vi "Add Acyclic Frame Triggers in Section.vi"(8 "error in":errorcluster, 10 "acyclic frames":T1[](array[typedef]), 11 "acyclic frames section":T2=18446744073709551615 format="%.0x") -> (0 "error out":errorcluster, 3 "acyclic frames section out":T2=18446744073709551615 format="%.0x")   [LabVIEW 2020, in "AIM MIL-STD-1553 Scripting.lvlib"]
doc: "Adds an Acyclic Frame Trigger for each element in <b>acyclic frames</b> to the <b>acyclic frames section</b>."
uses:
  AIM MIL-STD-1553 Scripting.lvlib
  <vilib>/NI VeriStand/Custom Device API/Custom Device Item Ref.ctl
  Constants.vi
  <vilib>/NI VeriStand/Custom Device API/Custom Device API.lvlib
  Shared/Acyclic Frame Definition.ctl
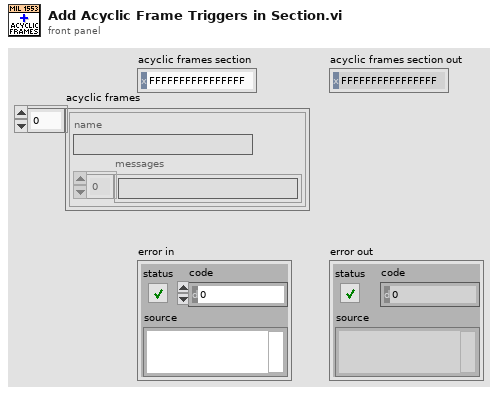
[diagram p1: front panel]
types:
  T1 = typedef "Acyclic Frame Definition.ctl" = cluster{"name":string, "messages":string[]}
  T2 = typedef "Custom Device API.lvlib/Custom Device Item Ref.ctl" = u64
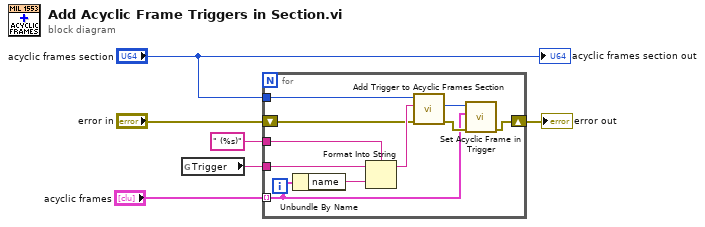
[diagram p0: block diagram]
diagram:
  n1 = global read "Constants.vi" "Trigger"() -> (w6:string)
  n2 = for {
    tunnel: w6 -> [w16]
    tunnel: " (%s)" ("format string") -> [w15]
    shift-right: [w10] -> w4
    shift-left: "error in" -> [w13]
    tunnel: "acyclic frames" -> [w7] mode=indexing
    tunnel: "acyclic frames section" -> [w12]
    n3 = Unbundle By Name(w7) -> ("name"=w8:string)
    n4 = Format Into String(format string=w15, initial string=w16, w8) -> (resulting string=w14:string)  [unwired: 1 in, 1 out]
    n5 = call "Add Trigger to Acyclic Frames Section.vi"("error in"=w13, "trigger name"=w14, "acyclic frames section"=w12) -> ("error out"=w11:errorcluster, "acyclic frame trigger"=w9:T2)  [unwired: 6 in, 1 out]
    n6 = call "Set Acyclic Frame in Trigger.vi"("error in"=w11, "acyclic frame"=w7, "acyclic frame trigger"=w9) -> ("error out"=w10:errorcluster)  [unwired: 7 in, 1 out]
  }
  "error out" <- w4
  "acyclic frames section out" <- "acyclic frames section"
